vi "DefaultFromIni.vi"(8 "error in (no error)":errorcluster, 11 "PacificPowerSource":refnum<class "PacificPowerSource.lvclass">) -> (0 "error out":errorcluster, 3 "PacificPowerSource":refnum<class "PacificPowerSource.lvclass">)   [LabVIEW 2018, in "AcPwrPlugins.lvlib" / "PacificPowerSource.lvclass"]
doc: "This VI reads the properties from the INI file and puts them into the LabVIEW class for further use."
uses:
  PacificPowerSource.lvclass
  C:/Program Files (x86)/National Instruments/LabVIEW 2018/user.lib/NIST/BaseClasses/BasePlugin_class/BasePlugin.lvclass
  TypeDefs/DeviceSettings.ctl
  TypeDefs/Measurements.ctl
  <userlib>/NIST/BaseClasses/BasePlugin_class/BasePlugin.lvclass/BasePlugin.ctl
  <userlib>/NIST/BaseClasses/BasePlugin_class/Accessors/Read PluginIniFilePath.vi
  AcPwrBaseClass/AcPwrBase.lvclass
  <vilib>/Utility/config.llb/NI_LVConfig.lvlib
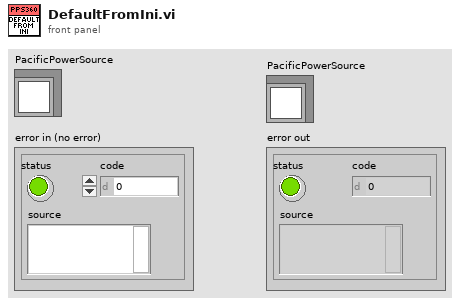
[diagram p1: front panel]
types:
  T1 = typedef "AcPwrPlugins.lvlib/PacificPowerSource.lvclass/Measurements.ctl" = cluster{"Handle":string, "Name":string, "Enabled ":bool, "Measurement Value":dbl, "Channel Name":enum16{"A", "B", "C"}, "Measurement Type ":enum16{"Voltage RMS L-N", "Voltage RMS L-L", "Frequency", "Current RMS", "Current Peak", "Crest Factor", "Power Factor", "Power VA", "Real Power"}}[]
  T2 = typedef "AcPwrPlugins.lvlib/PacificPowerSource.lvclass/DeviceSettings.ctl" = cluster{"Handle":string, "Connected":bool, "Clear Device (F)":bool, "btnIdQuery":bool, "btnReset":bool, "Program #":cluster{"Phase B (Degrees)":i32, "Waveform A (1: Sine)":i32, "Voltage Level (Va)":dbl, "Program Number (0)":i32, "Voltage Level (Vb) ":dbl, "Form (3: Three)":u16, "Coupling  (0: Direct)":u16, "Frequency (45Hz)":dbl, "Current Limit (40A)":dbl, "Phase C (Degrees)":i32, "Voltage Level (Vc)":dbl, "Waveform B (1: Sine)":i32, "Waveform C (1: Sine)":i32}[], "Impedance Parameters (off, 0.00)":cluster{"State":bool, "Impedance":dbl}, "Transient Execution (F)":bool, "OutputEnabled":bool, "Source Range":cluster{"Frequency Minimum (45 Hz)":dbl, "Frequency Maximum (1200 Hz)":dbl, "Voltage Maximum (V)":dbl, "Voltage Minimum (V)":dbl, "Range Control (0: Auto)":u16, "Initial Voltage (0V)":u16, "Frequency Range (600Hz)":u16}, "Port Type":enum16{"GPIB", "Serial"}}[]
  T3 = typedef "NI_LVConfig.lvlib/Config Data RefNum.ctl" = refnum<k1>
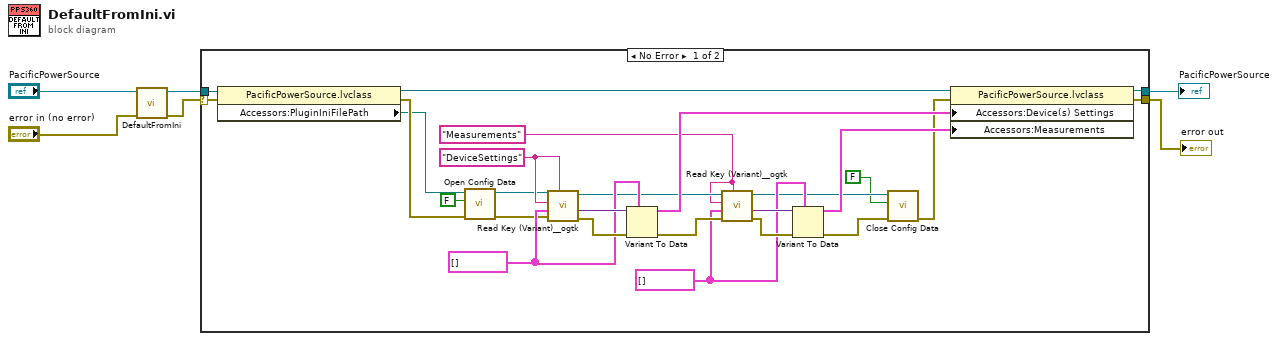
[diagram p0: block diagram]
diagram:
  n1 = call-parent "DefaultFromIni.vi"("error in (no error)"="error in (no error)", "AcPwrBase"="PacificPowerSource") -> ("error out"=w1:errorcluster, "AcPwrBase"=w2:refnum<class "PacificPowerSource.lvclass">)  [unwired: 8 in]
  n2 = case shown="No Error" w1 {
    selector: w1 -> [w31 w33]
    tunnel: [w27 w33] -> w6
    tunnel: [w28 w34] -> w5
    tunnel: w2 -> [w32 w34]
    frame No Error {
      w15 = "Measurements" ("section")
      w14 = T1 [] ("Measurements")
      w18 = T2 [] ("Load Settings")
      w19 = "DeviceSettings" ("section")
      n3 = property class="PacificPowerSource.lvclass"(reference=w32, error in=w31) -> (reference out=w29:refnum<class "PacificPowerSource.lvclass">, error out=w30:errorcluster, "Accessors:PluginIniFilePath"=w26:path)
      n4 = call <vilib>:"Open Config Data.vi"("error in (no error)"=w30, "create file if necessary (T)"=FALSE, "configuration file path"=w26) -> ("error out"=w8:errorcluster, "refnum"=w7:T3)  [unwired: 6 in, 1 out]
      n5 = call <userlib>:"Read Key (Variant)__ogtk.vi"("section"=w19, "error in (no error)"=w8, "type"=w18, "key (optional)"=w19, "refnum"=w7) -> ("error out"=w23:errorcluster, "key-value"=w24:variant, "refnum out"=w16:T3)  [unwired: 3 in, 1 out]
      n6 = Variant To Data(error in=w23, type=w18, Variant=w24) -> (data=w17:T2, error out=w20:errorcluster)
      n7 = call <userlib>:"Read Key (Variant)__ogtk.vi"("section"=w15, "error in (no error)"=w20, "type"=w14, "key (optional)"=w15, "refnum"=w16) -> ("error out"=w22:errorcluster, "key-value"=w21:variant, "refnum out"=w11:T3)  [unwired: 3 in, 1 out]
      n8 = Variant To Data(error in=w22, type=w14, Variant=w21) -> (data=w13:T1, error out=w12:errorcluster)
      n9 = call <vilib>:"Close Config Data.vi"("error in (no error)"=w12, "write file if changed (T)"=FALSE, "refnum"=w11) -> ("error out"=w10:errorcluster)  [unwired: 7 in, 1 out]
      n10 = property class="PacificPowerSource.lvclass"(reference=w29, error in=w10, "Accessors:Device(s) Settings"=w17, "Accessors:Measurements"=w13) -> (reference out=w28:refnum<class "PacificPowerSource.lvclass">, error out=w27:errorcluster)
    }
    frame Error {
    }
  }
  "error out" <- w6
  "PacificPowerSource" <- w5
